vi "CSet_Catalog.vi"(8 "error in (no error)":errorcluster, 11 "NetA_AgNA in":refnum<class "NetA_AgNA.lvclass">) -> (0 "error out":errorcluster, 1 "Cal Set Count":i32, 2 "Cal Set List":string[](array[string]), 3 "NetA_AgNA out":refnum<class "NetA_AgNA.lvclass">, 4 "Raw Dir List":string)   [LabVIEW 2014, in "NetA_AgNA.lvclass"]
doc: "Returns a list of proprietary cal set files (located in the Keysight folders)."
uses:
  NetA_AgNA.lvclass
  NetA_AgNA.lvclass/NetA_AgNA.ctl
  data/Agilent NA.lvlib
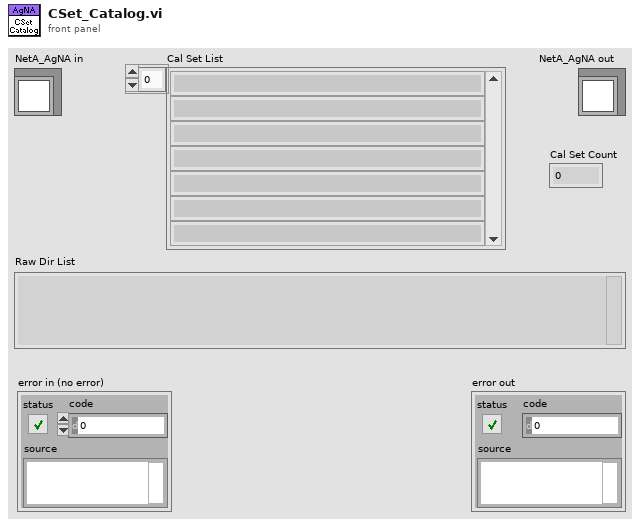
[diagram p1: front panel]
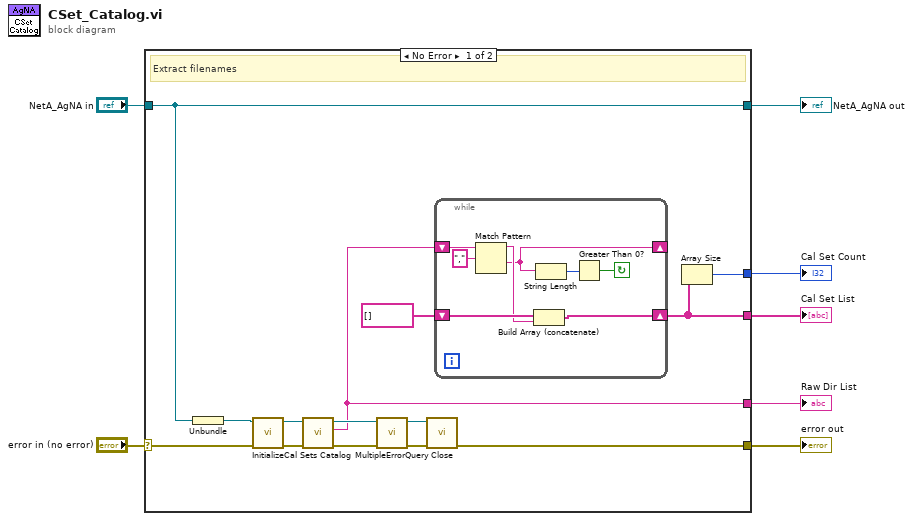
[diagram p0: block diagram]
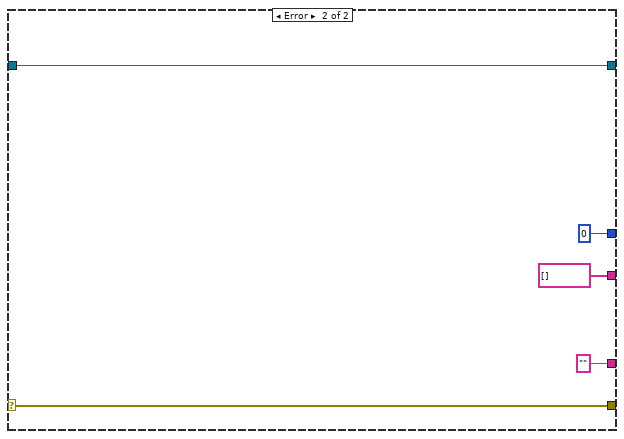
[diagram p2: hidden frame]
diagram:
  n1 = case shown="No Error" "error in (no error)" {
    selector: "error in (no error)" -> [w18 w33]
    tunnel: [w20 string[] []] -> w7
    tunnel: [w19 0] -> w6
    tunnel: [w15 w33] -> w4
    tunnel: [w10 "" ("Val")] -> w3
    tunnel: "NetA_AgNA in" -> [w9 w34]
    tunnel: [w9 w34] -> w1
    frame No Error {
      # "Extract filenames"
      n2 = Unbundle(w9) -> (w8:refnum<k15>)
      n3 = call "Initialize.vi"("error in (no error)"=w18, "resource name"=w8) -> ("error out"=w17:errorcluster, "instrument handle out"=w16:refnum<k15>)  [unwired: 8 in]
      n4 = call "Cal Sets Catalog.vi"("error in (no error)"=w17, "instrument handle"=w16) -> ("error out"=w14:errorcluster, "Val"=w10:string, "instrument handle out"=w13:refnum<k15>)  [unwired: 7 in]
      n5 = call "MultipleErrorQuery.vi"("error in (no error)"=w14, "instrument handle"=w13) -> ("error out"=w12:errorcluster, "instrument handle out"=w11:refnum<k15>)  [unwired: 7 in, 1 out]
      n6 = call "Close.vi"("error in (no error)"=w12, "instrument handle"=w11) -> ("error out"=w15:errorcluster)  [unwired: 9 in]
      n7 = while {
        shift-right: [w29] -> w20
        shift-left: string[] [] -> [w28]
        shift-right: [w24] -> _
        shift-left: w10 -> [w26]
        stop <- w22 continue-if-true
        n8 = Match Pattern(string=w26, regular expression=",") -> (before substring=w25:string, after substring=w24:string)  [unwired: 1 in, 2 out]
        n9 = Build Array (concatenate)(w28, w25) -> (w29:string[])
        n10 = String Length(string=w24) -> (length=w23:i32)
        n11 = Greater Than 0?(x=w23) -> (x > 0?=w22:bool)
      }
      n12 = Array Size(array=w20) -> (size(s)=w19:i32)
    }
    frame Error {
    }
  }
  "Raw Dir List" <- w3
  "error out" <- w4
  "Cal Set List" <- w7
  "Cal Set Count" <- w6
  "NetA_AgNA out" <- w1
